vi "PH_PILS.vis HVroomLockKnob.vi"(0 "i ref in":refnum<vi>, 5 "error IO":errorcluster) -> (14 "i ref out":refnum<vi>, 19 "error out":errorcluster)   [LabVIEW 2014, in "PH_PILS.lvlib"]
uses:
  PH_PILS.lvlib
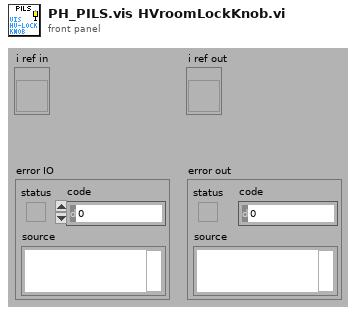
[diagram p1: front panel]
types:
  T1 = typedef "PH_PILS.lvlib/PH_PILS.i attribute.ctl" = cluster{"Boolean":cluster{"GUI Ref":refnum<vi>, "Status":i32}[], "GUI Refs Exp. Shutters":cluster{"1":refnum<vi>, "2":refnum<vi>, "3":refnum<vi>, "4":refnum<vi>}, "Tristate2Run GUI Refs":refnum<vi>[], "EO-Likes":cluster{"GUI Ref":refnum<vi>, "Status":i32}[], "Operation Mode":cluster{"Operation Mode":T2, "GUI":cluster{"Ref State":refnum<vi>, "Ref":refnum<vi>}, "Servicemode":cluster{"Tagname":string, "Status":i32}, "Labormode":cluster{"Tagname":string, "Status":i32}, "Searchmode":cluster{"Tagname":string, "Status":i32}, "Shotmode":cluster{"Tagname":string, "Status":i32}}, "Submode":cluster{"Submode":T3, "GUI":cluster{"Ref State":refnum<vi>, "Ref":refnum<vi>}, "Submode":cluster{"Tagname":string, "Status":i32}}, "Experiment":cluster{"Experiment":enum16{"unknown", "intern", "4 (Z6)", "3", "2", "1"}, "GUI":cluster{"Ref State":refnum<vi>, "Ref":refnum<vi>}, "intern":cluster{"Tagname":string, "Status":i32}, "Exp 4":cluster{"Tagname":string, "Status":i32}, "Exp 3":cluster{"Tagname":string, "Status":i32}, "Exp 2":cluster{"Tagname":string, "Status":i32}, "Exp 1":cluster{"Tagname":string, "Status":i32}}, "TristateNormal":cluster{"GUI Ref":refnum<vi>, "Status":i32}[], "Door Tags":cluster{"GUI Ref":refnum<vi>, "Status":i32}[], "GUIlessTags":cluster{"Name":string, "Status":i32}[], "Beamline GUI Refs":refnum<vi>[], "Special Boolean":cluster{"GUI Ref":refnum<vi>, "Status":i32}[], "Laserpower":cluster{"GUI Ref":refnum<vi>, "Status":i32}[], "Shutter":cluster{"GUI Ref":refnum<vi>, "Status":i32}[], "Tristate EO Like":cluster{"GUI Ref":refnum<vi>, "Status":i32}[], "PP":cluster{"GUI Ref":refnum<vi>, "Status":i32, "Head Ref":refnum<vi>, "Slider Ref":refnum<vi>}[], "Switch Knobs":cluster{"GUI Ref":refnum<vi>, "Status":i32}[], "Latch Knob GUI Refs":refnum<vi>[], "FailureCounter":i32, "Enabled Status":cluster{"Laser":i32, "PreAmp":i32, "MainAmp":i32}, "Mercury":refnum<vi>, "Instance Rods":string, "Logfile":path, "Beckhoff-Instance Internal":string, "Beckhoff-Instance External":string, "Enabling Rights":cluster{"Name":string, "Password":string, "PA?":bool, "MA?":bool, "Exp?":bool}[]}
  T2 = typedef "PH_PILS.lvlib/PH_PILS.Operation Mode.ctl" = enum16{"unknown", "Service", "Labor", "Search", "Shot"}
  T3 = typedef "PH_PILS.lvlib/PH_PILS.Submode.ctl" = enum16{"unknown", "HV-Normal", "HV-Test"}
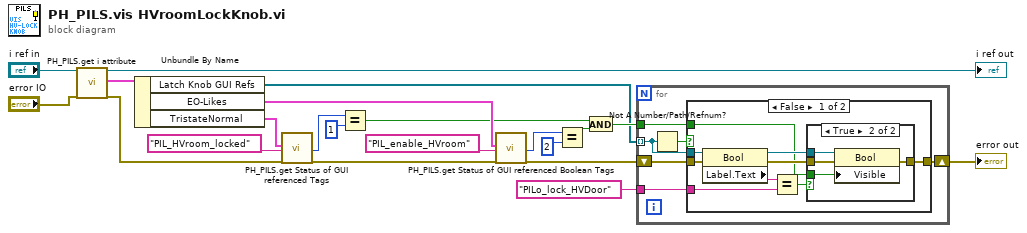
[diagram p0: block diagram]
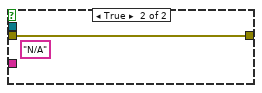
[diagram p3: hidden frame]
diagram:
  n1 = call "PH_PILS.get i attribute.vi"("i ref in"="i ref in", "error in (no error)"="error IO") -> ("i ref out"=→"i ref out":refnum<vi>, "i attribute"=w18:T1, "error out"=w3:errorcluster)  [unwired: 15 in]
  n2 = Unbundle By Name(w18) -> ("Latch Knob GUI Refs"=w5:refnum<vi>[], "EO-Likes"=w14:cluster{"GUI Ref":refnum<vi>, "Status":i32}[], "TristateNormal"=w1:cluster{"GUI Ref":refnum<vi>, "Status":i32}[])
  n3 = call "PH_PILS.get Status of GUI referenced Tags.vi"("Tags"=w1, "Tagname"="PIL_HVroom_locked", "error in"=w3) -> ("Status"=w11:i32, "error out"=w2:errorcluster)  [unwired: 13 in, 2 out]
  n4 = Equal?(x=w11, y=1) -> (x = y?=w6:bool)
  n5 = call "PH_PILS.get Status of GUI referenced Boolean Tags.vi"("Tags"=w14, "Tagname"="PIL_enable_HVroom", "error in"=w2) -> ("Status"=w10:i32, "error out"=w4:errorcluster)  [unwired: 13 in, 2 out]
  n6 = Equal?(x=w10, y=2) -> (x = y?=w7:bool)
  n7 = And(x=w6, y=w7) -> (x .and. y?=w15:bool)
  n8 = for {
    tunnel: w5 -> [w24] mode=indexing
    shift-right: [w25] -> w16
    shift-left: w4 -> [w27]
    tunnel: "PILo_lock_HVDoor" -> [w23]
    tunnel: w15 -> [w22]
    n9 = Not A Number/Path/Refnum?(number/path/refnum=w24) -> (NaN/Path/Refnum?=w26:bool)
    n10 = case shown="False" w26 {
      tunnel: w24 -> [w36 _]
      tunnel: w27 -> [w35 w42]
      tunnel: [w31 w42] -> w25
      tunnel: w23 -> [w33 _]
      tunnel: w22 -> [w28 _]
      frame False {
        n11 = property class="Bool"(reference=w36, error in=w35) -> (reference out=w30:refnum<vi>, error out=w32:errorcluster, "Label.Text"=w34:string)
        n12 = Equal?(x=w34, y=w33) -> (x = y?=w29:bool)
        n13 = case shown="True" w29 {
          tunnel: w32 -> [w37 w41]
          tunnel: [w37 w40] -> w31
          tunnel: w30 -> [_ w39]
          tunnel: w28 -> [_ w38]
          frame False {
          }
          frame True {
            n14 = property class="Bool"(reference=w39, error in=w41, "Visible"=w38) -> (error out=w40:errorcluster)  [unwired: 1 out]
          }
        }
      }
      frame True {
        (unwired) "N/A" ("Label.Text")
      }
    }
  }
  "error out" <- w16
